vi "SVG Parser.vi"(3 "error in (no error)":errorcluster, 5 "XML File Path":path) -> (0 "error out":errorcluster, 1 "Parsing Data":T5, 2 "Image Size":cluster{"Width":dbl, "Height":dbl})   [LabVIEW 2019]
doc: "This VI parses an SVG file using LabVIEW's built-in XML parser. It outputs the objects found in an SVG file as well as the canvas width and height."
uses:
  typedefs/Parsed Path - Cluster.ctl
  <vilib>/Analysis/Matrix/Datatypes/RealMatrix.ctl
  typedefs/Parsed Funnel - Cluster.ctl
  typedefs/Parsed Rect - Cluster.ctl
  <vilib>/Analysis/Matrix/NI_Matrix.lvlib
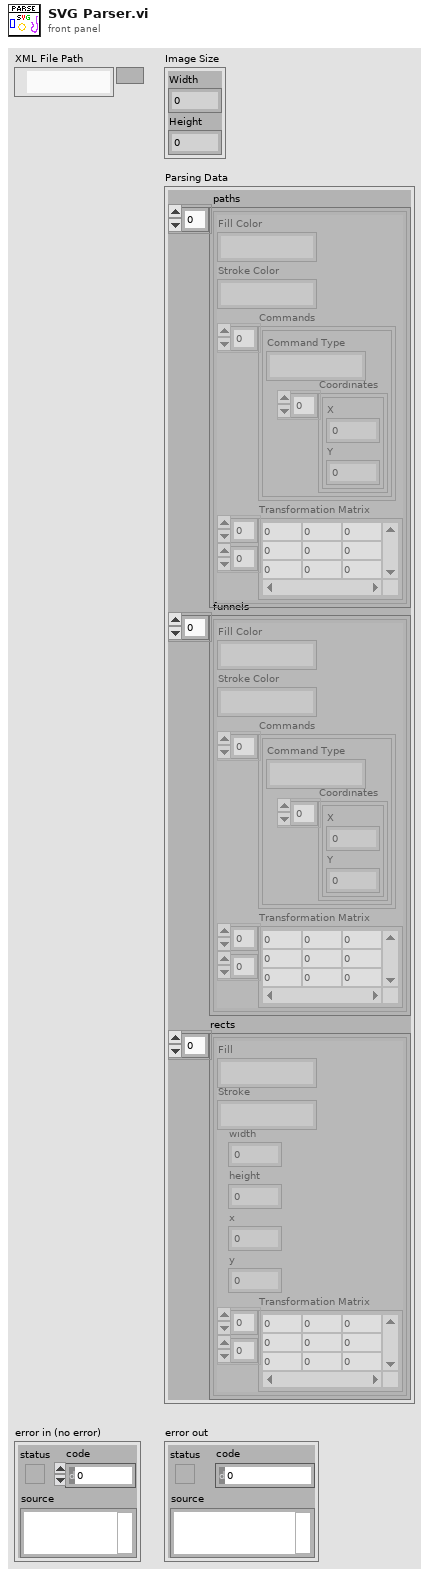
[diagram p1: front panel]
types:
  T1 = typedef "Parsed Path - Cluster.ctl" = cluster{"Fill Color":string, "Stroke Color":string, "Commands":cluster{"Command Type":string, "Coordinates":cluster{"X":dbl, "Y":dbl}[]}[], "Transformation Matrix":T2}
  T2 = typedef "NI_Matrix.lvlib/RealMatrix.ctl" = dbl[][]
  T3 = typedef "Parsed Funnel - Cluster.ctl" = cluster{"Fill Color":string, "Stroke Color":string, "Commands":cluster{"Command Type":string, "Coordinates":cluster{"X":dbl, "Y":dbl}[]}[], "Transformation Matrix":T2}
  T4 = typedef "Parsed Rect - Cluster.ctl" = cluster{"Fill":string, "Stroke":string, "width":dbl, "height":dbl, "x":dbl, "y":dbl, "Transformation Matrix":T2}
  T5 = cluster{" paths":T1[], " funnels":T3[], "rects":T4[]}
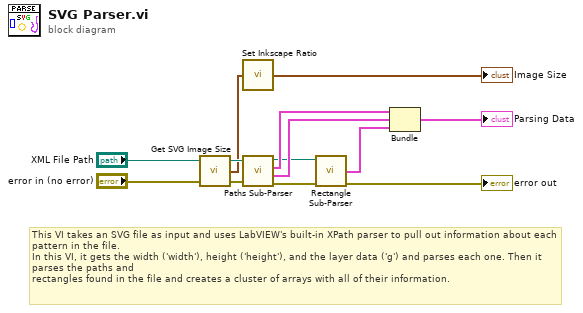
[diagram p0: block diagram]
diagram:
  # "This VI takes an SVG file as input and uses LabVIEW's built-in XPath parser to pull out information about each pattern in the file. \nIn this VI, it gets the width ('width'), height ('height'), and the layer data ('g') and parses each one. Then it parses the paths and \nrectangles found in the file and creates a cluster of arrays with all of their information."
  n1 = call "Get SVG Image Size.vi"("error in (no error)"="error in (no error)", "XML File Path In"="XML File Path") -> ("error out"=w7:errorcluster, "Image Size"=w6:cluster{"Width":dbl, "Height":dbl}, "XML File Path Out"=w8:path)  [unwired: 1 in]
  n2 = call "Set Inkscape Ratio.vi"("Image Size In"=w6) -> ("Image Size Out"=→"Image Size":cluster{"Width":dbl, "Height":dbl})
  n3 = call "Paths Sub-Parser.vi"("XML File Path In"=w8, "error in (no error)"=w7) -> ("XML File Path Out"=w2:path, "paths"=w4:T1[], "funnels"=w3:T3[], "error out"=w5:errorcluster)  [unwired: 1 in]
  n4 = call "Rectangle Sub-Parser.vi"("error in (no error)"=w5, "XML File Path In"=w2) -> ("error out"=→"error out":errorcluster, "rects"=w1:T4[])  [unwired: 1 in, 1 out]
  n5 = Bundle("paths"=w4, "funnels"=w3, "rects"=w1) -> (→"Parsing Data":T5)  [unwired: 1 in]
